vi "Load and display single image.vi"(0 "Image file path":path) -> (1 "Image":T2(plugin-control), 2 "Load image error":errorcluster)   [LabVIEW 2015]
panel:
  out "Image Type":T1 items=["Grayscale (U8)", "Grayscale (I16)", "Grayscale (SGL)", "Complex (CSG)", "RGB (U32)", "HSL (U32)", "RGB (U64)", "Grayscale (U16)"]
  out "File Data Type (bpp)":i32(ring)=3 items=["1 bit", "2 bits", "4 bits", "8 bits", "12 bits (unsigned)", "16 bits (unsigned)", "16 bits (signed)", "16 bits (RGB chunky)", "24 bits (RGB chunky)", "24 bits (RGB planar)", "32 bits (unsigned)", "32 bits (signed)", "32 bits (RGB chunky)", "32 bits (float)", "48 bits (Complex 2x24 int)", "64 bits (Complex 2x32 float)", "reserved", "24 bits (HSL)", "48 bits (RGB chunky)", "64 bits (RGB chunky)"]
  out "Image size (pixels)":string
  # "PN 23/12/2014"
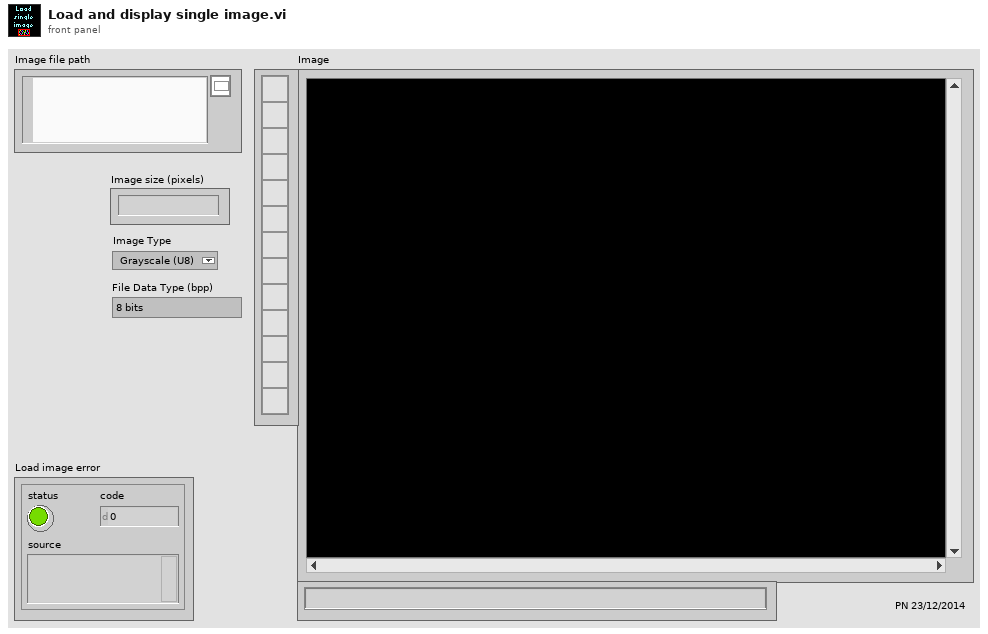
[diagram p1: front panel]
types:
  T1 = typedef "Image Type" = u32
  T2 = typedef "IMAQ Image.ctl" = refnum<image>
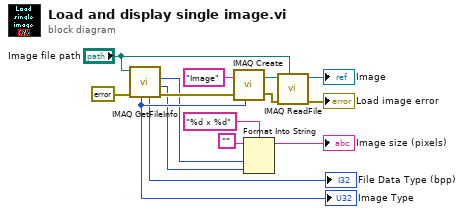
[diagram p0: block diagram]
diagram:
  n1 = call "IMAQ GetFileInfo"("error in (no error)"=errorcluster {"status"=FALSE, "code"=0, "source"=""} ("error in"), "File Path"="Image file path") -> ("error out"=w7:errorcluster, "Y Resolution"=w5:i32, "X Resolution"=w6:i32, "File Data Type"=→"File Data Type (bpp)":i32, "Image Type"=w8:T1)  [unwired: 3 in, 2 out]
  "Image Type" <- w8
  n2 = call "IMAQ Create"("Image Name"="Image", "Image Type"=w8, "error in (no error)"=w7) -> ("New Image"=w14:T2, "error out"=w13:errorcluster)  [unwired: 2 in]
  n3 = Format Into String(format string="%d x %d", initial string="", w6, w5) -> (resulting string=→"Image size (pixels)":string)  [unwired: 1 in, 1 out]
  n4 = call "IMAQ ReadFile"("File Path"="Image file path", "error in (no error)"=w13, "Image"=w14) -> ("error out"=→"Load image error":errorcluster, "Image Out"=→"Image":T2)  [unwired: 4 in, 3 out]
